vi "sig gpos.vi"() -> ()   [LabVIEW 2020]
uses:
  <vilib>/Analysis/Matrix/Datatypes/RealMatrix.ctl
  <vilib>/Analysis/Matrix/Numeric/Conversions/Array To Matrix - RA.vi
  <vilib>/Utility/file.llb/Write Delimited Spreadsheet (I64).vi
  <vilib>/Analysis/Matrix/NI_Matrix.lvlib
panel:
  out "overall time":u32
  in  "timing data out":path
  out "product":T1
  in  "vector size":i32=20
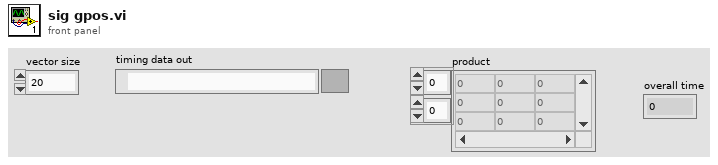
[diagram p1: front panel]
types:
  T1 = typedef "NI_Matrix.lvlib/RealMatrix.ctl" = dbl[][]
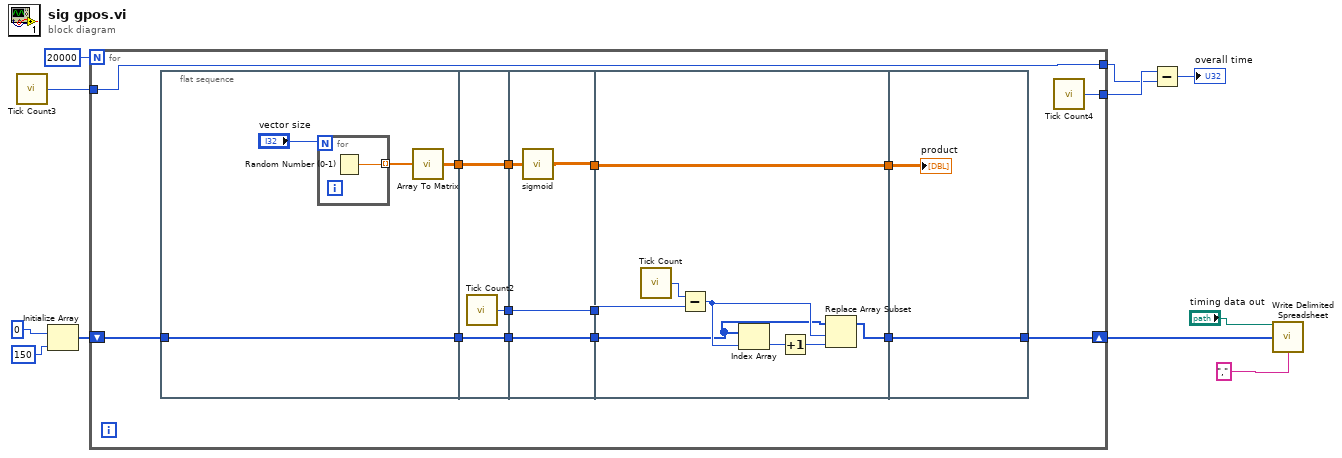
[diagram p0: block diagram]
diagram:
  n1 = call "Tick Count3"() -> ("Tick Count(uSec)"=w4:u32)
  n2 = Initialize Array(0, 150) -> (w8:i32[])
  n3 = for {
    N: 20000 -> [_]
    shift-right: [w14] -> w5
    shift-left: w8 -> [w16]
    tunnel: [w13] -> w2
    tunnel: w4 -> [w13]
    tunnel: [w12] -> w3
    n4 = flat-sequence {
      tunnel: [w28] -> w25
      tunnel: [w26] -> w17
      tunnel: w16 -> [w26]
      tunnel: w25 -> [w33]
      tunnel: [w33] -> w24
      tunnel: [w32] -> w23
      tunnel: [w31] -> w18
      tunnel: w17 -> [w31]
      tunnel: w24 -> [w34]
      tunnel: w23 -> [w37]
      tunnel: [w37] -> w22
      tunnel: [w35] -> w21
      tunnel: [w36] -> w19
      tunnel: w18 -> [w36]
      tunnel: w21 -> [w43]
      tunnel: w22 -> [w44]
      tunnel: [w43] -> w20
      tunnel: w19 -> [w39]
      tunnel: [w38] -> w15
      tunnel: w20 -> [w47]
      tunnel: w15 -> [w46]
      tunnel: [w46] -> w14
      frame #0 {
        n5 = for {
          N: "vector size" -> [_]
          tunnel: [w30] -> w29 mode=indexing
          n6 = Random Number (0-1)() -> (number: 0 to 1=w30:dbl)
        }
        n7 = call-poly <vilib>:"Array To Matrix.vi"("Real 1D Array"=w29) -> ("Real Matrix (Column Vector)"=w28:T1)
      }
      frame #1 {
        n8 = call "Tick Count2"() -> ("Tick Count(uSec)"=w32:u32)
      }
      frame #2 {
        n9 = call <vilib>:"sigmoid.vi"("x"=w34) -> ("y"=w35:T1)
      }
      frame #3 {
        n10 = call "Tick Count"() -> ("Tick Count(uSec)"=w45:u32)
        n11 = Subtract(x=w45, y=w44) -> (x-y=w40:u32)
        n12 = Index Array(array=w39, index=w40) -> (element=w41:i32)
        n13 = Increment(x=w41) -> (x+1=w42:i32)
        n14 = Replace Array Subset(array=w39, new element=w42, index=w40) -> (w38:i32[])
      }
      frame #4 {
        "product" <- w47
      }
    }
    n15 = call "Tick Count4"() -> ("Tick Count(uSec)"=w12:u32)
  }
  n16 = Subtract(x=w3, y=w2) -> (x-y=→"overall time":u32)
  n17 = call-poly <vilib>:"Write Delimited Spreadsheet.vi"("file path (dialog if empty)"="timing data out", "1D data"=w5, "delimiter (\\t)"=",") -> ()  [unwired: 11 in, 2 out]
